vi "Ramp to Speed with Constant Acceleration.vi"(7 "Time Between Points (ms)":dbl, 8 "Error In":errorcluster, 9 "Acceleration (in/s2)":dbl, 10 "Final Speed (in/s)":dbl, 11 "Initial Snapshot":T2) -> (0 "Error Out":errorcluster, 1 "Duration (s)":dbl, 2 "Motion Profile Portion":T1[](array[typedef]), 3 "Final Snapshot":T2, 4 "Distance (in)":dbl)   [LabVIEW 2019, in "Motion Profile Generator.lvclass"]
uses:
  Motion Profile Generator.lvclass
  Type Defs/Motion Snapshot.ctl
  Type Defs/Motion Profile Point.ctl
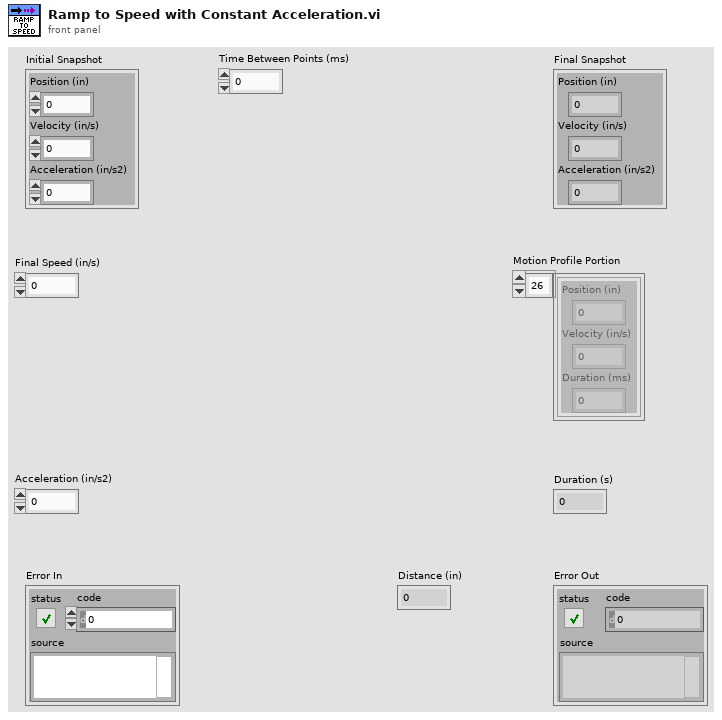
[diagram p1: front panel]
types:
  T1 = typedef "Motion Profile Generator.lvclass/Motion Profile Point.ctl" = cluster{"Position (in)":dbl, "Velocity (in/s)":dbl, "Duration (ms)":dbl}
  T2 = typedef "Motion Profile Generator.lvclass/Motion Snapshot.ctl" = cluster{"Position (in)":dbl, "Velocity (in/s)":dbl, "Acceleration (in/s2)":dbl}
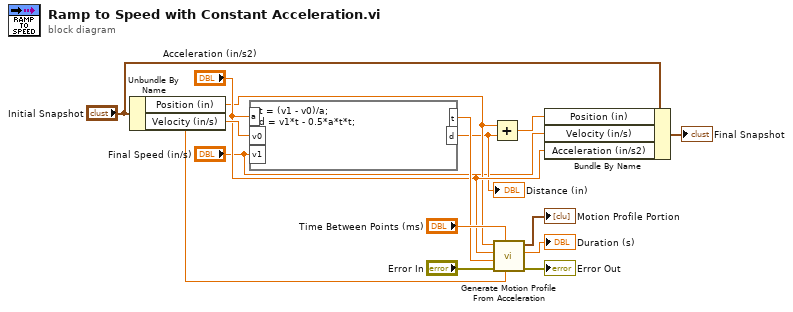
[diagram p0: block diagram]
diagram:
  n1 = Unbundle By Name("Initial Snapshot") -> ("Position (in)"=w4:dbl, "Velocity (in/s)"=w10:dbl)
  n2 = formula code="t = (v1 - v0)/a;\nd = v1*t - 0.5*a*t*t;"("a"="Acceleration (in/s2)", "v0"=w10, "v1"="Final Speed (in/s)") -> ("d"=w3:dbl, "t"=w11:dbl)
  "Distance (in)" <- w3
  n3 = Add(x=w4, y=w3) -> (x+y=w2:dbl)
  n4 = call "Generate Motion Profile From Acceleration.vi"("Initial Velocity (in/s)"=w10, "Time Between Points (ms)"="Time Between Points (ms)", "Error In"="Error In", "Movement Duration (s)"=w11, "Acceleration (in/s2)"="Acceleration (in/s2)", "Initial Position (in)"=w4) -> ("Error Out"=→"Error Out":errorcluster, "Duration (s)"=→"Duration (s)":dbl, "Motion Profile Portion"=→"Motion Profile Portion":T1[])  [unwired: 3 in]
  n5 = Bundle By Name(cluster="Initial Snapshot", "Position (in)"=w2, "Velocity (in/s)"="Final Speed (in/s)", "Acceleration (in/s2)"="Acceleration (in/s2)") -> (→"Final Snapshot":T2)
